vi "Interface connect.vi"(8 "error in":errorcluster, 11 "interface in":refnum<class "Network Interface.lvclass">) -> (0 "error out":errorcluster, 3 "interface out":refnum<class "Network Interface.lvclass">)   [LabVIEW 2021, in "Network Interface.lvclass"]
doc: "This provides an interface for reading from a network bus."
uses:
  Network Interface.lvclass
  Network Interface.lvclass/Network Interface.ctl
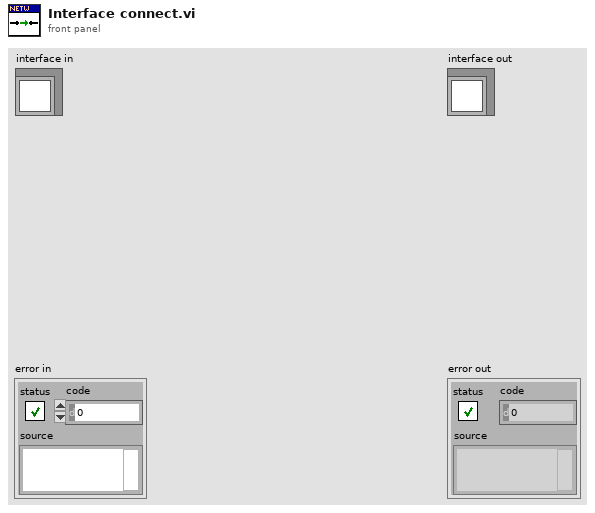
[diagram p1: front panel]
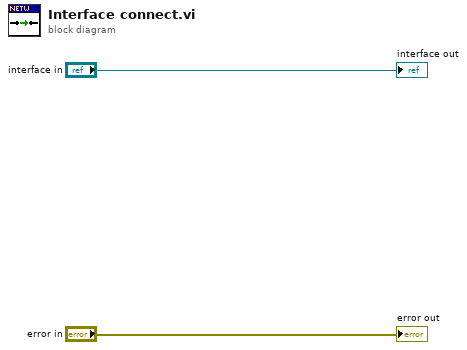
[diagram p0: block diagram]
diagram:
  "error out" <- "error in"
  "interface out" <- "interface in"
